vi "Write tdms file ref.vi"(8 "error in":errorcluster, 10 "tdms file ref":refnum<k34>, 11 "Report Viewer in":refnum<class "Report Viewer.lvclass">) -> (0 "error out":errorcluster, 3 "Report Viewer out":refnum<class "Report Viewer.lvclass">)   [LabVIEW 2019, in "Report Viewer.lvlib" / "Report Viewer.lvclass"]
uses:
  Library/Report Viewer.lvclass
  Library/Report Viewer.lvclass/Report Viewer.ctl
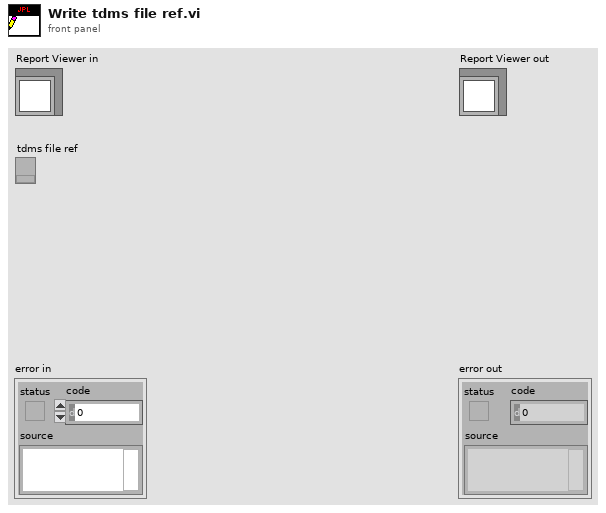
[diagram p1: front panel]
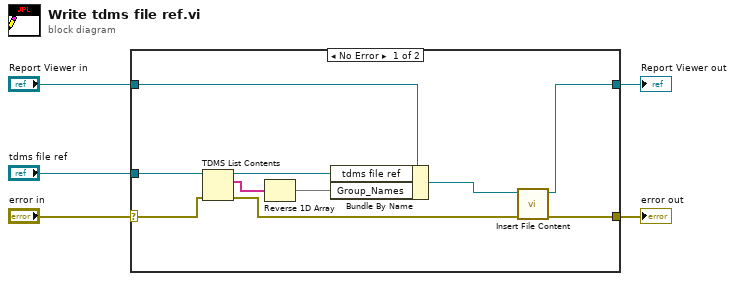
[diagram p0: block diagram]
diagram:
  n1 = case shown="No Error" "error in" {
    selector: "error in" -> [w12 w16]
    tunnel: [w9 w16] -> w4
    tunnel: [w7 w17] -> w2
    tunnel: "Report Viewer in" -> [w15 w17]
    tunnel: "tdms file ref" -> [w14 _]
    frame No Error {
      n2 = TDMS List Contents(4:w12, 7:w14) -> (0:w10:errorcluster, 2:w11:string[], 3:w13:refnum<k34>)  [unwired: 1 in, 1 out]
      n3 = Reverse 1D Array(array=w11) -> (reversed array=w6:string[])
      n4 = Bundle By Name(cluster=w15, "tdms file ref"=w13, "Group_Names"=w6) -> (w8:refnum<class "Report Viewer.lvclass">)
      n5 = call "Insert File Content.vi"("error in"=w10, "Report Viewer in"=w8) -> ("error out"=w9:errorcluster, "Report Viewer out"=w7:refnum<class "Report Viewer.lvclass">)  [unwired: 8 in]
    }
    frame Error {
    }
  }
  "error out" <- w4
  "Report Viewer out" <- w2
